vi "get text between brackets.vi"(10 "Python String":string) -> (2 "Text Between Brakets":string)   [LabVIEW 2020, in "jki_python_data_tools.lvlib"]
uses:
  jki_python_data_tools.lvlib
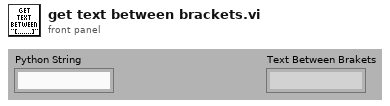
[diagram p1: front panel]
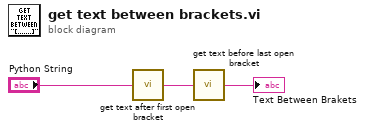
[diagram p0: block diagram]
diagram:
  n1 = call "get text after first open bracket.vi"("Python String"="Python String") -> ("Text After First Open Bracket"=w3:string)
  n2 = call "get text before last open bracket.vi"("Python String"=w3) -> ("Text After Last Open Bracket"=→"Text Between Brakets":string)
